vi "DisplayPanel.vi"() -> ()   [LabVIEW 2013]
uses:
  MvLVLib/MvCameraControl.lvlib
  MvLVLib/VIs/CreateGigEHandle.vi
  MvLVLib/VIs/CreateU3VHandle.vi
panel:
  out "GenTLDeviceArray":T1(array[cluster])
  out "Image":T2(plugin-control)
  out "U3VDeviceArray":T3(array[cluster])
  out "GigEDeviceArray":T4(array[cluster])
  in  "pConvertInfo In":T5
  out "PixelFormat":u32
  out "handle out":u64
  in  "handle":u64
  out "PayloadSize":u32
  out "pFrameInfoEx out":T6
  out "nHeight":u32
  out "nWidth":u32
  out "Acquisision Flag":bool
  in  "Trigger Mode":bool
  in  "Continuous":bool
  out "打开标志":bool
  in  "stop":bool
  in  "Trigger Once":bool
  in  "Stop":bool
  in  "Start":bool
  in  "Open Device":bool
  in  "Close Device":bool
  in  "error in (no error) 2":errorcluster caption="错误输入（无错误）"
  in  "Refresh Devices":bool
  in  "Device List":u16(ring)
  # "Initialize"
  # "Acquisition"
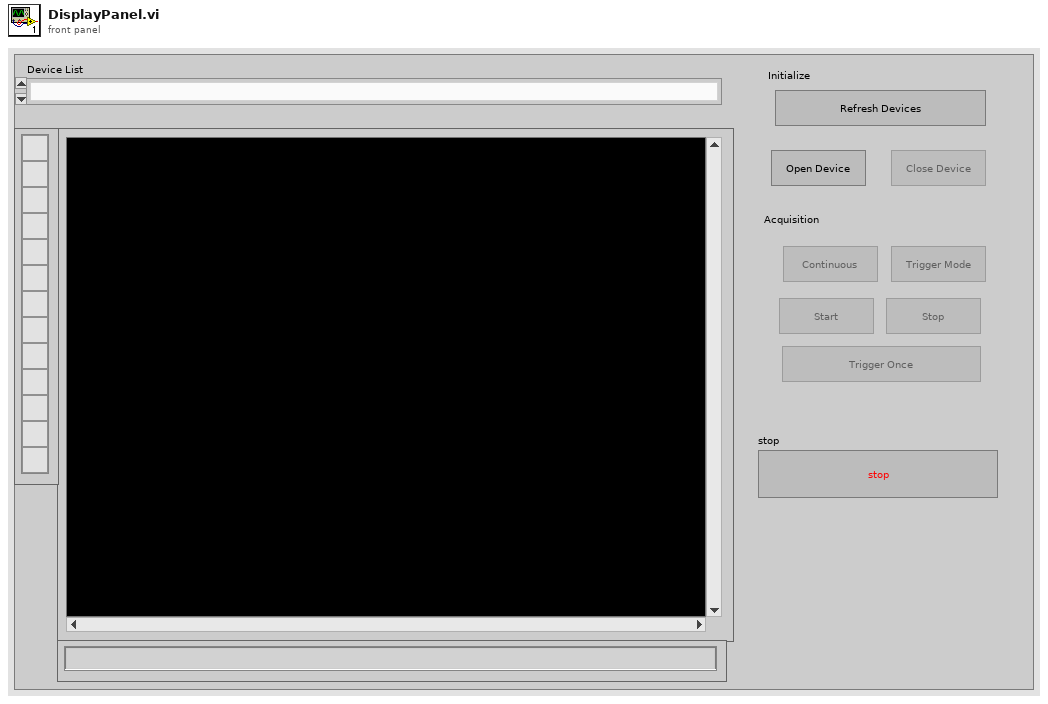
[diagram p1: front panel]
types:
  T1 = cluster{"nMajorVer":u16, "nMinorVer":u16, "nMacAddrHigh":u32, "nMacAddrLow":u32, "nTLayerType":u32, "nReserved0":u32, "nReserved1":u32, "nReserved2":u32, "nReserved3":u32, "chInterfaceID":string, "chVendorName":string, "chModelName":string, "chManufacturerInfo":string, "chDeviceVersion":string, "chSerialNumber":string, "chUserDefinedName":string, "chDeviceID":string, "nRes0":u32, "nRes1":u32, "nRes2":u32, "nRes3":u32, "nRes4":u32, "nRes5":u32, "nRes6":u32}[]
  T2 = typedef "IMAQ Image.ctl" = refnum<image>
  T3 = cluster{"nMajorVer":u16, "nMinorVer":u16, "nMacAddrHigh":u32, "nMacAddrLow":u32, "nTLayerType":u32, "nReserved0":u32, "nReserved1":u32, "nReserved2":u32, "nReserved3":u32, "CrtlInEndPoint":u8, "CrtlOutEndPoint":u8, "StreamEndPoint":u8, "EventEndPoint":u8, "idVendor":u16, "idProduct":u16, "nDeviceNumber":u32, "chDeviceGUID":string, "chVendorName":string, "chModelName":string, "chFamilyName":string, "chDeviceVersion":string, "chManufacturerName":string, "chSerialNumber":string, "chUserDefinedName":string, "nbcdUSB":u32, "nDeviceAddress":u32, "nRes0":u32, "nRes1":u32, "nResAlign":u32}[]
  T4 = cluster{"nMajorVer":u16, "nMinorVer":u16, "nMacAddrHigh":u32, "nMacAddrLow":u32, "nTLayerType":u32, "nReserved0":u32, "nReserved1":u32, "nReserved2":u32, "nReserved3":u32, "nIpCfgOption":u32, "nIpCfgCurrent":u32, "nCurrentIp":u32, "nCurrentSubNetMask":u32, "nDefaultGateWay":u32, "chManualfacturerName":string, "chModelName":string, "chDeviceVersion":string, "chManufacturerSpecificInfo":string, "chSerialNumber":string, "chUserDefinedName":string, "nNetExport":u32, "nRes0":u32, "nRes1":u32, "nRes2":u32, "nRes3":u32}[]
  T5 = cluster{"nWidth":u16, "nHeight":u16, "enSrcPixelType":u32, "nSrcDataLen":u32, "enDstPixelType":u32, "nDstLen":u32, "nDstBufferSize":u32, "nRes0":u32, "nRes1":u32, "nRes2":u32, "nRes3":u32}
  T6 = cluster{"nWidth":u16, "nHeight":u16, "enPixelType":i32, "nFrameNum":u32, "nDevTimeStampHigh":u32, "nDevTimeStampLow":u32, "nReserved0":u32, "nHostTimeStamp":i64, "nFrameLen":u32, "nSecondCount]":u32, "nCycleCount":u32, "nCycleOffset":u32, "fGain":u32, "fExposureTime":u32, "nAverageBrightness":u32, "nRed":u32, "nGreen":u32, "nBlue":u32, "nFrameCounter":u32, "nTriggerIndex":u32, "nInput":u32, "nOutput":u32, "nOffsetX":u32, "nOffsetY":u32, "nReserved[0]":u32, "nReserved[1]":u32, "nReserved[2]":u32, "nReserved[3]":u32, "nReserved[4]":u32, "nReserved[5]":u32, "nReserved[6]":u32, "nReserved[7]":u32, "nReserved[8]":u32, "nReserved[9]":u32, "nReserved[10]":u32, "nReserved[11]":u32, "nReserved[12]":u32, "nReserved[13]":u32, "nReserved[14] 10":u32, "nReserved[15] 11":u32, "nReserved[16] 12":u32, "nReserved[17] 13":u32, "nReserved[18] 14":u32, "nReserved[19] 15":u32, "nReserved[20] 16":u32, "nReserved[21] 17":u32, "nReserved[22] 18":u32, "nReserved[23] 19":u32, "nReserved[24] 20":u32, "nReserved[25] 21":u32, "nReserved[26] 22":u32, "nReserved[27] 23":u32, "nReserved[28] 24":u32, "nReserved[29] 25":u32, "nReserved[30] 26":u32, "nReserved[31] 27":u32, "nReserved[32] 28":u32, "nReserved[33] 29":u32, "nReserved[34] 30":u32, "nReserved[35] 31":u32, "nReserved[36] 32":u32, "nReserved[37] 33":u32, "nReserved[38] 34":u32, "nReserved[39] 35":u32, "nReserved[40] 36":u32}
  T7 = enum8{"Enabled", "Disabled", "Disabled and Grayed Out"}
  T8 = cluster{"nCurValue":u32, "nMax":u32, "nMin":u32, "nInc":u32, "nReserved[0]":u32, "nReserved[1]":u32, "nReserved[2]":u32, "nReserved[3]":u32}
  T9 = cluster{"nCurValue":u32, "nSupportedNum":u32, "nSupportValue":u32[], "nReserved[0]":u32, "nReserved[1]":u32, "nReserved[2]":u32, "nReserved[3]":u32}
  T10 = cluster{"nWidth":u32, "nHeight":u32, "enSrcPixelType":u32, "nSrcDataLen":u32, "enDstPixelType":u32, "nDstLen":u32, "nDstBufferSize":u32, "nRes0":u32, "nRes1":u32, "nRes2":u32, "nRes3":u32}
  T11 = typedef "Image Type" = u32
  T12 = cluster{"nMajorVer":u16, "nMinorVer":u16, "nMacAddrHigh":u32, "nMacAddrLow":u32, "nTLayerType":u32, "nReserved0":u32, "nReserved1":u32, "nReserved2":u32, "nReserved3":u32, "nIpCfgOption":u32, "nIpCfgCurrent":u32, "nCurrentIp":u32, "nCurrentSubNetMask":u32, "nDefaultGateWay":u32, "chManualfacturerName":string, "chModelName":string, "chDeviceVersion":string, "chManufacturerSpecificInfo":string, "chSerialNumber":string, "chUserDefinedName":string, "nNetExport":u32, "nRes0":u32, "nRes1":u32, "nRes2":u32, "nRes3":u32}
  T13 = cluster{"nMajorVer":u16, "nMinorVer":u16, "nMacAddrHigh":u32, "nMacAddrLow":u32, "nTLayerType":u32, "nReserved0":u32, "nReserved1":u32, "nReserved2":u32, "nReserved3":u32, "CrtlInEndPoint":u8, "CrtlOutEndPoint":u8, "StreamEndPoint":u8, "EventEndPoint":u8, "idVendor":u16, "idProduct":u16, "nDeviceNumber":u32, "chDeviceGUID":string, "chVendorName":string, "chModelName":string, "chFamilyName":string, "chDeviceVersion":string, "chManufacturerName":string, "chSerialNumber":string, "chUserDefinedName":string, "nbcdUSB":u32, "nDeviceAddress":u32, "nRes0":u32, "nRes1":u32, "nResAlign":u32}
  T14 = cluster{"nMajorVer":u16, "nMinorVer":u16, "nMacAddrHigh":u32, "nMacAddrLow":u32, "nTLayerType":u32, "nReserved0":u32, "nReserved1":u32, "nReserved2":u32, "nReserved3":u32, "chInterfaceID":string, "chVendorName":string, "chModelName":string, "chManufacturerInfo":string, "chDeviceVersion":string, "chSerialNumber":string, "chUserDefinedName":string, "chDeviceID":string, "nRes0":u32, "nRes1":u32, "nRes2":u32, "nRes3":u32, "nRes4":u32, "nRes5":u32, "nRes6":u32}
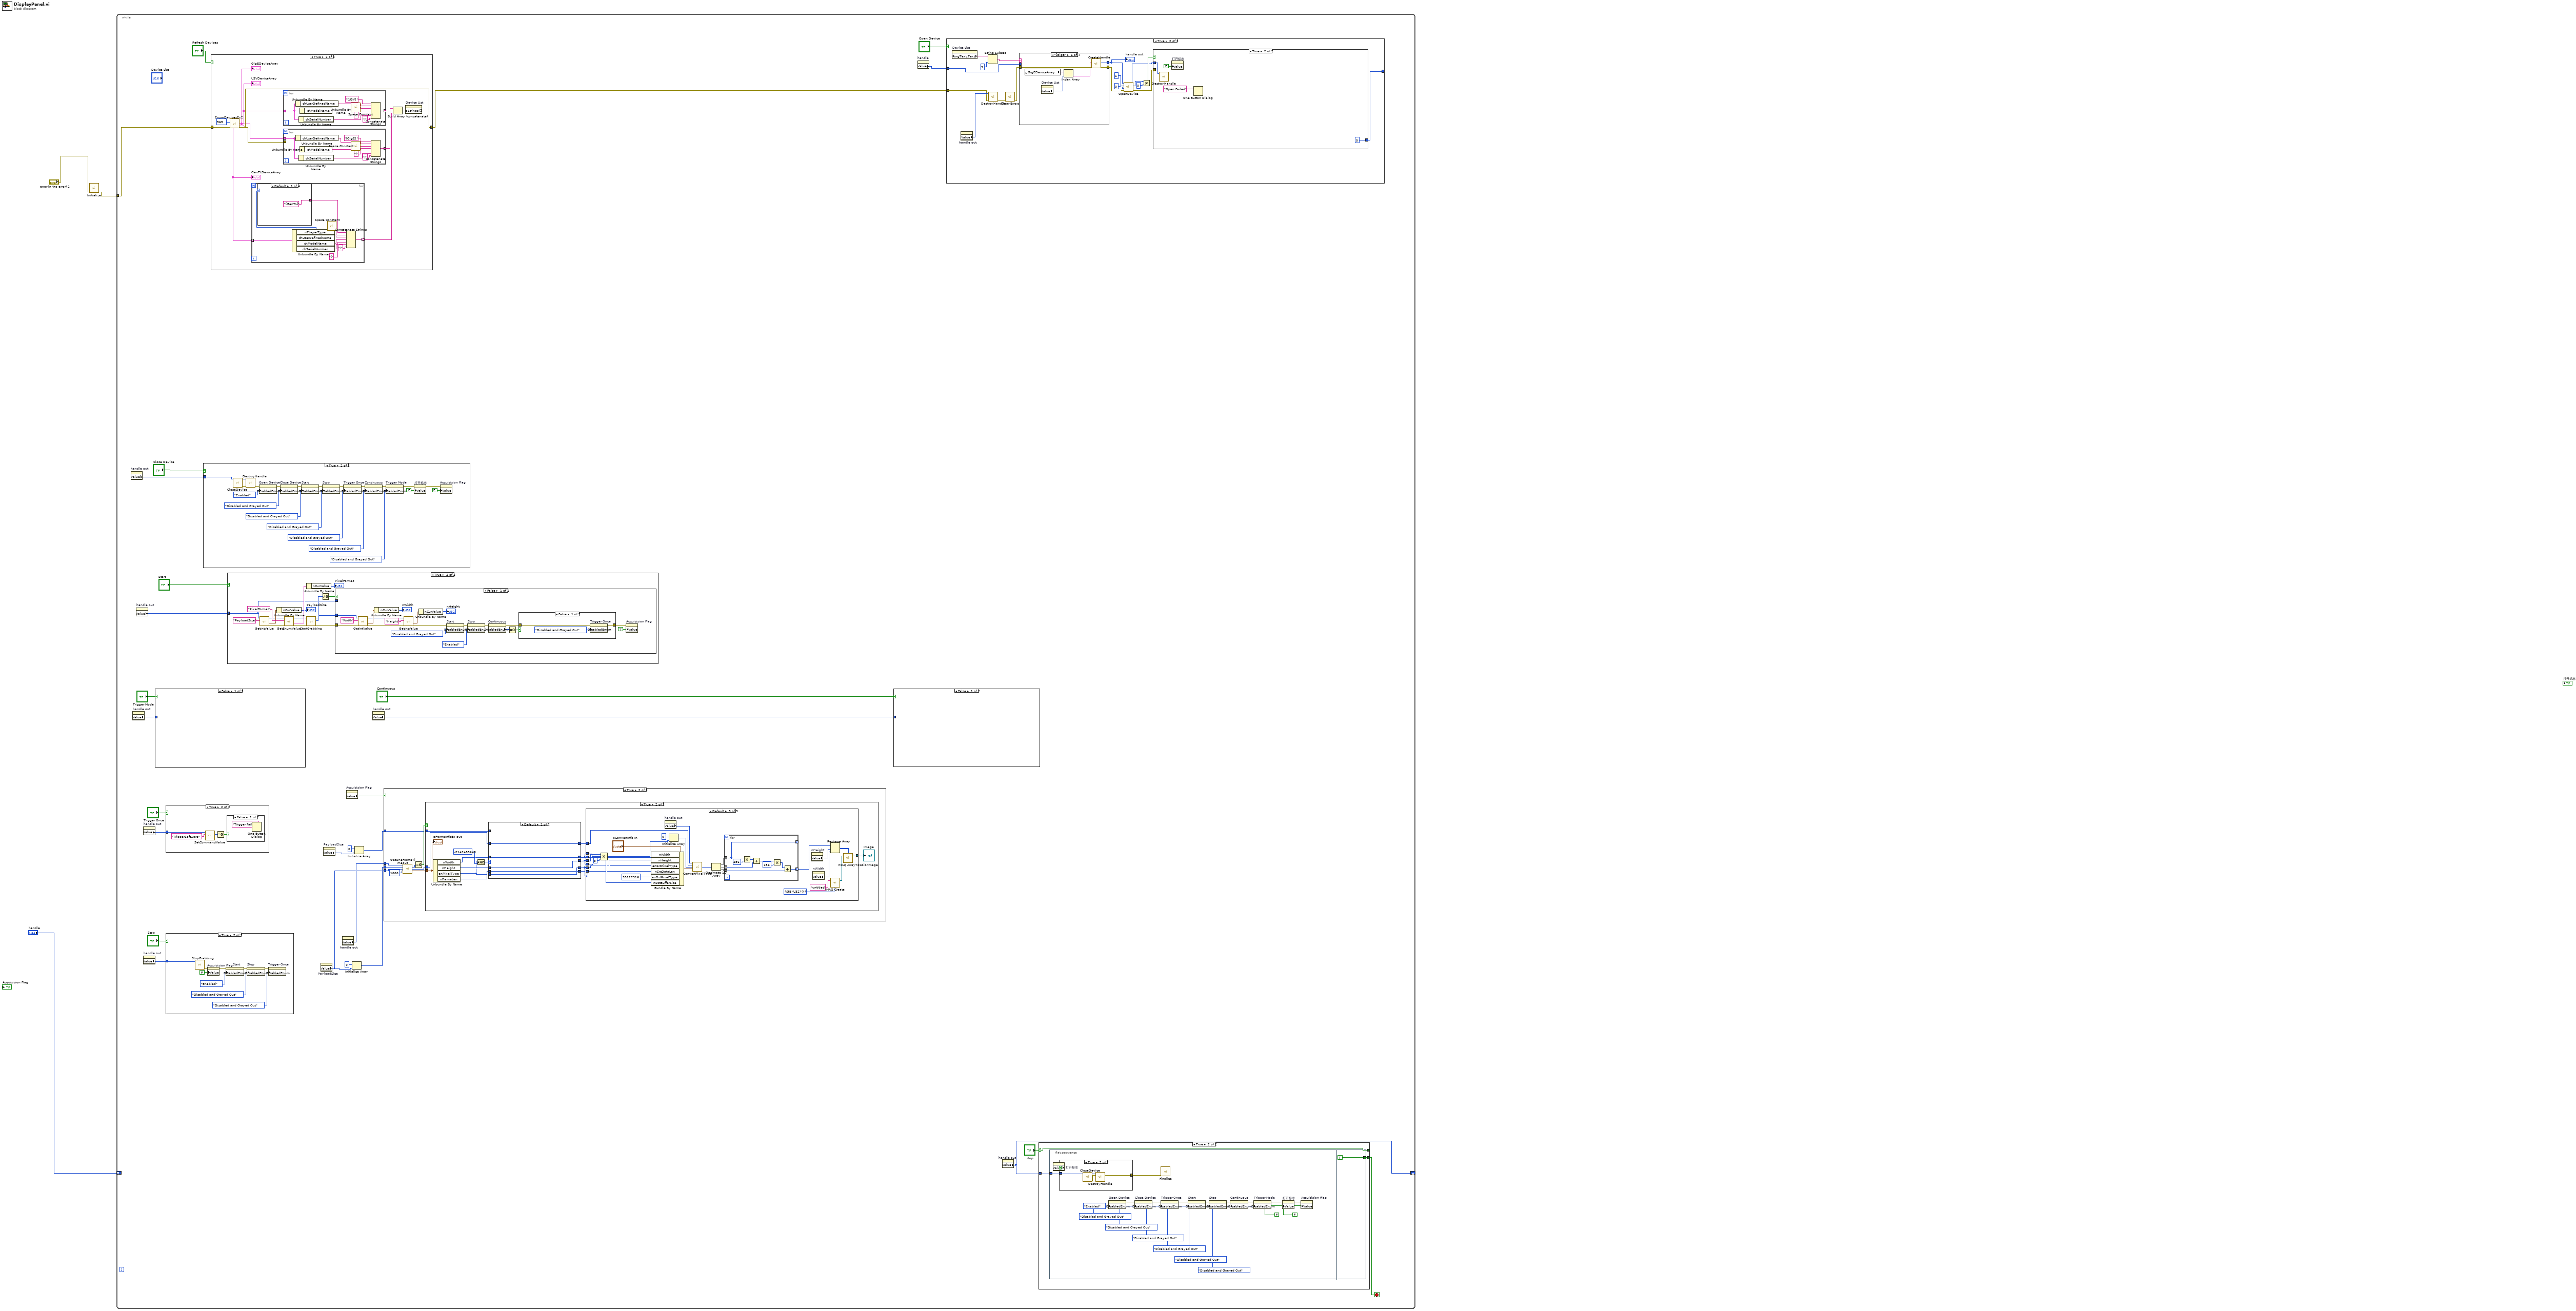
[diagram p0: block diagram]
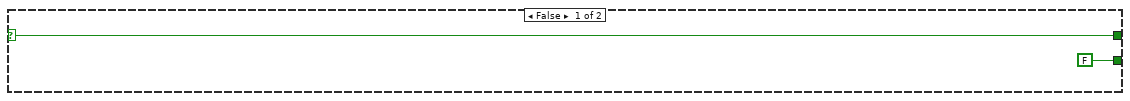
[diagram p2: hidden frame]
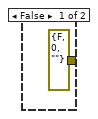
[diagram p3: hidden frame]
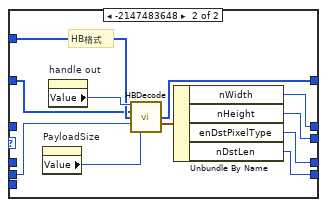
[diagram p6: hidden frame]
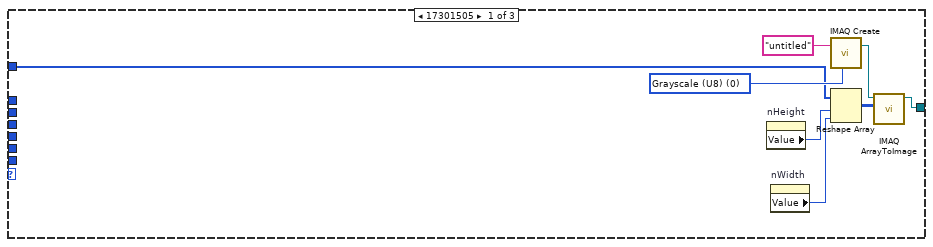
[diagram p7: hidden frame]
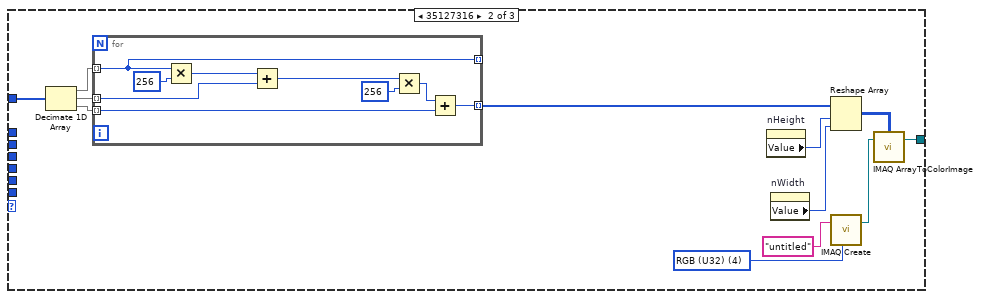
[diagram p8: hidden frame]
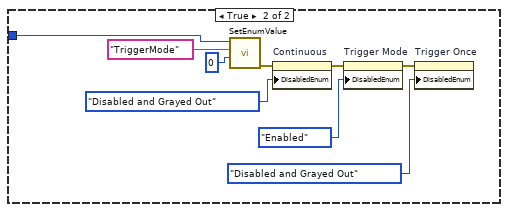
[diagram p10: hidden frame]
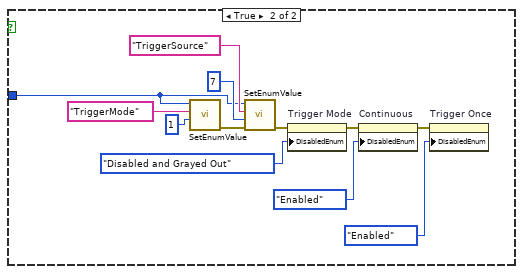
[diagram p11: hidden frame]
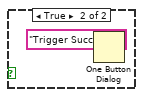
[diagram p13: hidden frame]
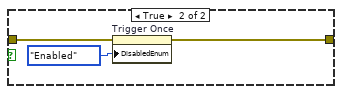
[diagram p15: hidden frame]
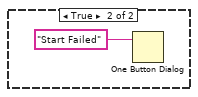
[diagram p16: hidden frame]
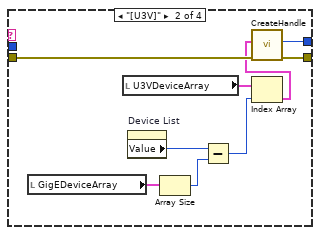
[diagram p19: hidden frame]
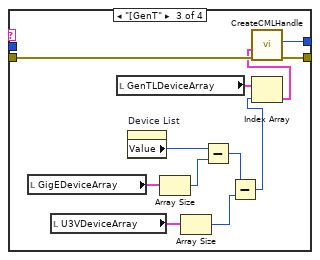
[diagram p20: hidden frame]
diagram:
  n1 = call "Initialize.vi"("error in (no error)"="error in (no error) 2") -> ("error out"=w2:errorcluster)  [unwired: 9 in, 1 out]
  n2 = while {
    shift-right: [w10] -> _
    shift-left: "handle" -> [_]
    tunnel: w2 -> [w11]
    stop <- w8 stop-if-true
    n3 = property on="handle out" class="DigNum (strict)"() -> ("Value"=w20:u64)  [unwired: 2 in, 2 out]
    n4 = property on="handle out" class="DigNum (strict)"() -> ("Value"=w15:u64)  [unwired: 2 in, 2 out]
    n5 = property on="handle out" class="DigNum (strict)"() -> ("Value"=w16:u64)  [unwired: 2 in, 2 out]
    n6 = property on="handle out" class="DigNum (strict)"() -> ("Value"=w19:u64)  [unwired: 2 in, 2 out]
    n7 = property on="handle out" class="DigNum (strict)"() -> ("Value"=w18:u64)  [unwired: 2 in, 2 out]
    n8 = case shown="False" "Trigger Mode" {
      tunnel: w15 -> [_ w186]
      frame False {
      }
      frame True {
        n9 = call "SetEnumValue.vi"("nValue"=u32 1, "strKey"="TriggerMode", "handle"=w186) -> ("error out"=w192:errorcluster)  [unwired: 6 in, 2 out]
        n10 = call "SetEnumValue.vi"("error in (no error)"=w192, "nValue"=u32 7, "strKey"="TriggerSource", "handle"=w186) -> ("error out"=w191:errorcluster)  [unwired: 5 in, 2 out]
        n11 = property on="Trigger Mode" class="Bool"(error in=w191, "DisabledEnum"=T7."Disabled and Grayed Out" ("禁用")) -> (error out=w190:errorcluster)  [unwired: 1 in, 1 out]
        n12 = property on="Continuous" class="Bool"(error in=w190, "DisabledEnum"=T7."Enabled" ("禁用")) -> (error out=w188:errorcluster)  [unwired: 1 in, 1 out]
        n13 = property on="Trigger Once" class="Bool"(error in=w188, "DisabledEnum"=T7."Enabled" ("禁用")) -> ()  [unwired: 1 in, 2 out]
      }
    }
    n14 = case shown="True" "Trigger Once" {
      tunnel: w19 -> [_ w201]
      frame False {
      }
      frame True {
        n15 = call "SetCommandValue.vi"("strValue"="TriggerSoftware", "handle"=w201) -> ("function return"=w199:i32)  [unwired: 7 in, 2 out]
        n16 = Equal To 0?(x=w199) -> (x = 0?=w198:bool)
        n17 = case shown="False" w198 {
          frame False {
            n18 = One Button Dialog(message="Trigger Failed") -> ()  [unwired: 1 in, 1 out]
          }
          frame True {
            n19 = One Button Dialog(message="Trigger Success") -> ()  [unwired: 1 in, 1 out]
          }
        }
      }
    }
    n20 = case shown="True" "Stop" {
      tunnel: w18 -> [_ w176]
      frame False {
      }
      frame True {
        n21 = call "StopGrabbing.vi"("handle"=w176) -> ("error out"=w175:errorcluster)  [unwired: 8 in, 2 out]
        n22 = property on="Acquisision Flag" class="Bool (strict)"(error in=w175, "Value"=FALSE ("采集标志")) -> (error out=w170:errorcluster)  [unwired: 1 in, 1 out]
        n23 = property on="Start" class="Bool"(error in=w170, "DisabledEnum"=T7."Enabled" ("禁用")) -> (error out=w169:errorcluster)  [unwired: 1 in, 1 out]
        n24 = property on="Stop" class="Bool"(error in=w169, "DisabledEnum"=T7."Disabled and Grayed Out" ("禁用")) -> (error out=w168:errorcluster)  [unwired: 1 in, 1 out]
        n25 = property on="Trigger Once" class="Bool"(error in=w168, "DisabledEnum"=T7."Disabled and Grayed Out" ("禁用")) -> ()  [unwired: 1 in, 2 out]
      }
    }
    n26 = case shown="True" "Close Device" {
      tunnel: w20 -> [_ w247]
      frame False {
      }
      frame True {
        n27 = call "CloseDevice.vi"("handle"=w247) -> ("error out"=w249:errorcluster, "handle out"=w246:u64)  [unwired: 8 in, 1 out]
        n28 = call "DestroyHandle.vi"("error in (no error)"=w249, "handle"=w246) -> ("error out"=w248:errorcluster)  [unwired: 8 in, 1 out]
        n29 = property on="Open Device" class="Bool"(error in=w248, "DisabledEnum"=T7."Enabled" ("禁用")) -> (error out=w262:errorcluster)  [unwired: 1 in, 1 out]
        n30 = property on="Close Device" class="Bool"(error in=w262, "DisabledEnum"=T7."Disabled and Grayed Out" ("禁用")) -> (error out=w261:errorcluster)  [unwired: 1 in, 1 out]
        n31 = property on="Start" class="Bool"(error in=w261, "DisabledEnum"=T7."Disabled and Grayed Out" ("禁用")) -> (error out=w260:errorcluster)  [unwired: 1 in, 1 out]
        n32 = property on="Stop" class="Bool"(error in=w260, "DisabledEnum"=T7."Disabled and Grayed Out" ("禁用")) -> (error out=w259:errorcluster)  [unwired: 1 in, 1 out]
        n33 = property on="Trigger Once" class="Bool"(error in=w259, "DisabledEnum"=T7."Disabled and Grayed Out" ("禁用")) -> (error out=w256:errorcluster)  [unwired: 1 in, 1 out]
        n34 = property on="Continuous" class="Bool"(error in=w256, "DisabledEnum"=T7."Disabled and Grayed Out" ("禁用")) -> (error out=w254:errorcluster)  [unwired: 1 in, 1 out]
        n35 = property on="Trigger Mode" class="Bool"(error in=w254, "DisabledEnum"=T7."Disabled and Grayed Out" ("禁用")) -> (error out=w253:errorcluster)  [unwired: 1 in, 1 out]
        n36 = property on="打开标志" class="Bool (strict)"(error in=w253, "Value"=FALSE ("打开标志")) -> (error out=w251:errorcluster)  [unwired: 1 in, 1 out]
        n37 = property on="Acquisision Flag" class="Bool (strict)"(error in=w251, "Value"=FALSE ("采集标志")) -> ()  [unwired: 1 in, 2 out]
      }
    }
    n38 = case shown="True" "Refresh Devices" {
      tunnel: [w335 w345] -> w22
      tunnel: w11 -> [w335 w344]
      frame False {
        n39 = property on="GigEDeviceArray" class="Arr (strict)" props=["Value"]() -> ()  [unwired: 2 in, 3 out]
        n40 = property on="U3VDeviceArray" class="Arr (strict)" props=["Value"]() -> ()  [unwired: 2 in, 3 out]
      }
      frame True {
        n41 = call "EnumDevicesEx2.vi"("nLayerType"=965, "error in (no error)"=w344) -> ("GigEDeviceArray"=w340:T4, "U3VDeviceArray"=w339:T3, "GenTLDevice"=w337:T1, "error out"=w345:errorcluster)  [unwired: 8 in, 2 out]
        "GigEDeviceArray" <- w340
        "U3VDeviceArray" <- w339
        "GenTLDeviceArray" <- w337
        n42 = for {
          tunnel: w337 -> [w352] mode=indexing
          tunnel: [w350] -> w336 mode=indexing
          n43 = Unbundle By Name(w352) -> ("nTLayerType"=w347:u32, "chUserDefinedName"=w355:string, "chModelName"=w349:string, "chSerialNumber"=w348:string)
          n44 = case shown="Default" w347 {
            tunnel: ["[GenTL]" ("字符串") "[GenTL CML]" ("字符串") "[GenTL CXP]" ("字符串") "[GenTL XOF]" ("字符串")] -> w346
            frame Default {
            }
            frame 128 {
            }
            frame 256 {
            }
            frame 512 {
            }
          }
          n45 = call <vilib>:"Space Constant.vi"() -> ("String"=w354:string)
          n46 = Concatenate Strings(w346, w355, w354, w349, "(" ("字符串"), w348, ")" ("字符串")) -> (w350:string)
        }
        n47 = for {
          tunnel: w339 -> [w364] mode=indexing
          tunnel: [w361] -> w342 mode=indexing
          n48 = Unbundle By Name(w364) -> ("chUserDefinedName"=w368:string)
          n49 = Unbundle By Name(w364) -> ("chSerialNumber"=w363:string)
          n50 = Unbundle By Name(w364) -> ("chModelName"=w366:string)
          n51 = call <vilib>:"Space Constant.vi"() -> ("String"=w367:string)
          n52 = Concatenate Strings("[U3V] " ("字符串"), w368, w367, w366, "(" ("字符串"), w363, ")" ("字符串")) -> (w361:string)
        }
        n53 = for {
          tunnel: w345 -> [_]
          tunnel: w340 -> [w371] mode=indexing
          tunnel: [w370] -> w343 mode=indexing
          n54 = Unbundle By Name(w371) -> ("chUserDefinedName"=w374:string)
          n55 = Unbundle By Name(w371) -> ("chSerialNumber"=w372:string)
          n56 = Unbundle By Name(w371) -> ("chModelName"=w373:string)
          n57 = call <vilib>:"Space Constant.vi"() -> ("String"=w377:string)
          n58 = Concatenate Strings("[GigE] " ("字符串"), w374, w377, w373, "(" ("字符串"), w372, ")" ("字符串")) -> (w370:string)
        }
        n59 = Build Array (concatenate)(w343, w342, w336) -> (w341:string[])
        n60 = property on="Device List" class="Ring (strict)"("Strings []"=w341) -> ()  [unwired: 2 in, 2 out]
      }
    }
    n61 = case shown="True" "Start" {
      tunnel: w16 -> [_ w208]
      frame False {
      }
      frame True {
        n62 = call "GetIntValue.vi"("strKey"="PayloadSize", "handle"=w208) -> ("error out"=w214:errorcluster, "pIntValue out"=w210:T8, "handle out"=w206:u64)  [unwired: 6 in, 1 out]
        n63 = Unbundle By Name(w210) -> ("nCurValue"=→"PayloadSize":u32)
        n64 = call "GetEnumValue.vi"("error in (no error)"=w214, "strKey"="PixelFormat", "handle"=w206) -> ("error out"=w213:errorcluster, "pEnumValue out"=w215:T9, "handle out"=w205:u64)  [unwired: 5 in, 1 out]
        n65 = Unbundle By Name(w215) -> ("nCurValue"=→"PixelFormat":u32)
        n66 = call "StartGrabbing.vi"("error in (no error)"=w213, "handle"=w205) -> ("error out"=w212:errorcluster, "function return"=w218:i32, "handle out"=w204:u64)  [unwired: 7 in]
        n67 = Not Equal To 0?(x=w218) -> (x != 0?=w217:bool)
        n68 = case shown="False" w217 {
          tunnel: w208 -> [_ _]
          tunnel: w212 -> [w221 _]
          tunnel: w204 -> [w220 _]
          frame False {
            n69 = call "GetIntValue.vi"("error in (no error)"=w221, "strKey"="Width", "handle"=w220) -> ("error out"=w228:errorcluster, "pIntValue out"=w222:T8, "handle out"=w219:u64)  [unwired: 5 in, 1 out]
            n70 = Unbundle By Name(w222) -> ("nCurValue"=→"nWidth":u32)
            n71 = call "GetIntValue.vi"("error in (no error)"=w228, "strKey"="Height", "handle"=w219) -> ("error out"=w227:errorcluster, "pIntValue out"=w225:T8)  [unwired: 5 in, 2 out]
            n72 = Unbundle By Name(w225) -> ("nCurValue"=→"nHeight":u32)
            n73 = property on="Start" class="Bool"(error in=w227, "DisabledEnum"=T7."Disabled and Grayed Out" ("禁用")) -> (error out=w237:errorcluster)  [unwired: 1 in, 1 out]
            n74 = property on="Stop" class="Bool"(error in=w237, "DisabledEnum"=T7."Enabled" ("禁用")) -> (error out=w223:errorcluster)  [unwired: 1 in, 1 out]
            n75 = property on="Continuous" class="Bool"(error in=w223) -> (error out=w233:errorcluster, "DisabledEnum"=w234:T7)  [unwired: 1 in, 1 out]
            n76 = Equal To 0?(x=w234) -> (x = 0?=w235:bool)
            n77 = case shown="False" w235 {
              tunnel: w233 -> [w240 w243]
              tunnel: [w239 w242] -> w232
              frame False {
                n78 = property on="Trigger Once" class="Bool"(error in=w240, "DisabledEnum"=T7."Disabled and Grayed Out" ("禁用")) -> (error out=w239:errorcluster)  [unwired: 1 in, 1 out]
              }
              frame True {
                n79 = property on="Trigger Once" class="Bool"(error in=w243, "DisabledEnum"=T7."Enabled" ("禁用")) -> (error out=w242:errorcluster)  [unwired: 1 in, 1 out]
              }
            }
            n80 = property on="Acquisision Flag" class="Bool (strict)"(error in=w232, "Value"=TRUE ("采集标志")) -> ()  [unwired: 1 in, 2 out]
          }
          frame True {
            n81 = One Button Dialog(message="Start Failed") -> ()  [unwired: 1 in, 1 out]
          }
        }
      }
    }
    n82 = property on="PayloadSize" class="DigNum (strict)"() -> ("Value"=w7:u32)  [unwired: 2 in, 2 out]
    n83 = property on="PayloadSize" class="DigNum (strict)"() -> ("Value"=w6:u32)  [unwired: 2 in, 2 out]
    n84 = property on="handle out" class="DigNum (strict)"() -> ("Value"=w17:u64)  [unwired: 2 in, 2 out]
    n85 = property on="Acquisision Flag" class="Bool (strict)"() -> ("Value"=w23:bool)  [unwired: 2 in, 2 out]
    n86 = Initialize Array(u8 0 ("元素"), w7) -> (w12:u8[])
    n87 = Initialize Array(u8 0 ("元素"), w6) -> (w4:u8[])
    n88 = property on="handle out" class="DigNum (strict)"() -> ("Value"=w14:u64)  [unwired: 2 in, 2 out]
    n89 = case shown="True" w23 {
      tunnel: w17 -> [_ w69]
      tunnel: w12 -> [_ w68]
      tunnel: w7 -> [_ w67]
      tunnel: w4 -> [_ w63]
      frame False {
      }
      frame True {
        n90 = call "GetOneFrameTimeout.vi"("handle"=w69, "pData"=w68, "nDataSize"=w67, "nMsec"=1000) -> ("function return"=w66:i32, "pData Out"=w65:u8[], "pFrameInfoEx out"=w64:T6)  [unwired: 7 in, 2 out]
        n91 = Equal To 0?(x=w66) -> (x = 0?=w71:bool)
        n92 = case shown="True" w71 {
          tunnel: w65 -> [_ w81]
          tunnel: w64 -> [_ w85]
          tunnel: w63 -> [_ w82]
          frame False {
          }
          frame True {
            n93 = Unbundle By Name(w85) -> ("nWidth"=w74:u16, "nHeight"=w73:u16, "enPixelType"=w72:i32, "nFrameLen"=w80:u32)
            n94 = Compound Arithmetic op=AND(w72, -2147483648 ("value")) -> (w83:i32)
            n95 = case shown="Default" w83 {
              tunnel: w82 -> [_ w101]
              tunnel: w81 -> [w91 w100]
              tunnel: w80 -> [w88 w99]
              tunnel: [w91 w96] -> w79
              tunnel: [w90 w95] -> w78
              tunnel: [w89 w94] -> w77
              tunnel: [w87 w93] -> w76
              tunnel: [w88 w92] -> w75
              tunnel: w74 -> [w90 _]
              tunnel: w73 -> [w89 _]
              tunnel: w72 -> [w87 _]
              frame Default {
              }
              frame -2147483648 {
                # "HB格式"
                n96 = property on="PayloadSize" class="DigNum (strict)"() -> ("Value"=w98:u32)  [unwired: 2 in, 2 out]
                n97 = property on="handle out" class="DigNum (strict)"() -> ("Value"=w102:u64)  [unwired: 2 in, 2 out]
                n98 = call "HBDecode.vi"("handle"=w102, "pSrcData"=w100, "pDstBuf In"=w101, "SrcDataLen"=w99, "DstBufferSize"=w98) -> ("pDstBuf Out"=w96:u8[], "pHBDecode Out"=w97:T10)  [unwired: 6 in, 3 out]
                n99 = Unbundle By Name(w97) -> ("nWidth"=w95:u32, "nHeight"=w94:u32, "enDstPixelType"=w93:u32, "nDstLen"=w92:u32)
              }
            }
            n100 = case shown="Default" w76 {
              tunnel: w79 -> [w103 w114 w132]
              tunnel: w77 -> [_ _ w153]
              tunnel: w78 -> [_ _ w152]
              tunnel: [w104 w113 w137] -> w86
              tunnel: w78 -> [_ _ w136]
              tunnel: w77 -> [_ _ w135]
              tunnel: w76 -> [_ _ w134]
              tunnel: w75 -> [_ _ w133]
              frame 17301505 {
                w110 = T11 0 items=["Grayscale (U8)", "Grayscale (I16)", "Grayscale (SGL)", "Complex (CSG)", "RGB (U32)", "HSL (U32)", "RGB (U64)", "Grayscale (U16)"] ("Image Type")
                n101 = property on="nHeight" class="DigNum (strict)"() -> ("Value"=w106:u32)  [unwired: 2 in, 2 out]
                n102 = property on="nWidth" class="DigNum (strict)"() -> ("Value"=w105:u32)  [unwired: 2 in, 2 out]
                n103 = call "IMAQ Create"("Image Name"="untitled", "Image Type"=w110) -> ("New Image"=w108:T2)  [unwired: 3 in, 1 out]
                n104 = Reshape Array(w103, w106, w105) -> (w107:u8[][])
                n105 = call "IMAQ ArrayToImage"("Image Pixels (U8)"=w107, "Image"=w108) -> ("Image Out"=w104:T2)  [unwired: 8 in, 1 out]
              }
              frame 35127316 {
                w122 = T11 4 items=["Grayscale (U8)", "Grayscale (I16)", "Grayscale (SGL)", "Complex (CSG)", "RGB (U32)", "HSL (U32)", "RGB (U64)", "Grayscale (U16)"] ("Image Type")
                n106 = Decimate 1D Array(w114) -> (w115:u8[], w116:u8[], w117:u8[])
                n107 = for {
                  tunnel: w115 -> [w123] mode=indexing
                  tunnel: w116 -> [w129] mode=indexing
                  tunnel: w117 -> [w125] mode=indexing
                  tunnel: [w124] -> w118 mode=indexing
                  tunnel: [w123] -> _ mode=indexing
                  n108 = Multiply(x=w123, y=256) -> (x*y=w130:i32)
                  n109 = Add(x=w130, y=w129) -> (x+y=w128:i32)
                  n110 = Multiply(x=w128, y=256) -> (x*y=w126:i32)
                  n111 = Add(x=w126, y=w125) -> (x+y=w124:i32)
                }
                n112 = property on="nHeight" class="DigNum (strict)"() -> ("Value"=w112:u32)  [unwired: 2 in, 2 out]
                n113 = property on="nWidth" class="DigNum (strict)"() -> ("Value"=w111:u32)  [unwired: 2 in, 2 out]
                n114 = Reshape Array(w118, w112, w111) -> (w119:i32[][])
                n115 = call "IMAQ Create"("Image Name"="untitled", "Image Type"=w122) -> ("New Image"=w120:T2)  [unwired: 3 in, 1 out]
                n116 = call "IMAQ ArrayToColorImage"("Image Pixels (U32)"=w119, "Image"=w120) -> ("Image Out"=w113:T2)  [unwired: 3 in, 1 out]
              }
              frame Default {
                w148 = T11 4 items=["Grayscale (U8)", "Grayscale (I16)", "Grayscale (SGL)", "Complex (CSG)", "RGB (U32)", "HSL (U32)", "RGB (U64)", "Grayscale (U16)"] ("Image Type")
                n117 = Compound Arithmetic op=MULTIPLY(w153, w152, u32 3 ("值")) -> (w150:u32)
                n118 = Bundle By Name(cluster="pConvertInfo In", "nWidth"=w136, "nHeight"=w135, "enSrcPixelType"=w134, "nSrcDataLen"=w133, "enDstPixelType"=u32 35127316, "nDstBufferSize"=w150) -> (w149:T5)
                n119 = property on="handle out" class="DigNum (strict)"() -> ("Value"=w156:u64)  [unwired: 2 in, 2 out]
                n120 = Initialize Array(u8 0 ("元素"), w150) -> (w155:u8[])
                n121 = call "ConvertPixelType.vi"("handle"=w156, "pSrcData"=w132, "pDstBuf In"=w155, "pConvertInfo In"=w149) -> ("pDstBuf Out"=w140:u8[])  [unwired: 7 in, 4 out]
                n122 = Decimate 1D Array(w140) -> (w141:u8[], w142:u8[], w143:u8[])
                n123 = for {
                  tunnel: w141 -> [w159] mode=indexing
                  tunnel: w142 -> [w165] mode=indexing
                  tunnel: w143 -> [w161] mode=indexing
                  tunnel: [w160] -> w144 mode=indexing
                  tunnel: [w159] -> _ mode=indexing
                  n124 = Multiply(x=w159, y=256) -> (x*y=w166:i32)
                  n125 = Add(x=w166, y=w165) -> (x+y=w164:i32)
                  n126 = Multiply(x=w164, y=256) -> (x*y=w162:i32)
                  n127 = Add(x=w162, y=w161) -> (x+y=w160:i32)
                }
                n128 = property on="nHeight" class="DigNum (strict)"() -> ("Value"=w139:u32)  [unwired: 2 in, 2 out]
                n129 = property on="nWidth" class="DigNum (strict)"() -> ("Value"=w138:u32)  [unwired: 2 in, 2 out]
                n130 = Reshape Array(w144, w139, w138) -> (w145:i32[][])
                n131 = call "IMAQ Create"("Image Name"="untitled", "Image Type"=w148) -> ("New Image"=w146:T2)  [unwired: 3 in, 1 out]
                n132 = call "IMAQ ArrayToColorImage"("Image Pixels (U32)"=w145, "Image"=w146) -> ("Image Out"=w137:T2)  [unwired: 3 in, 1 out]
              }
            }
            "Image" <- w86
            "pFrameInfoEx out" <- w85
          }
        }
      }
    }
    n133 = case shown="False" "Continuous" {
      tunnel: w14 -> [_ w177]
      frame False {
      }
      frame True {
        n134 = call "SetEnumValue.vi"("nValue"=u32 0, "strKey"="TriggerMode", "handle"=w177) -> ("error out"=w178:errorcluster)  [unwired: 6 in, 2 out]
        n135 = property on="Continuous" class="Bool"(error in=w178, "DisabledEnum"=T7."Disabled and Grayed Out" ("禁用")) -> (error out=w182:errorcluster)  [unwired: 1 in, 1 out]
        n136 = property on="Trigger Mode" class="Bool"(error in=w182, "DisabledEnum"=T7."Enabled" ("禁用")) -> (error out=w180:errorcluster)  [unwired: 1 in, 1 out]
        n137 = property on="Trigger Once" class="Bool"(error in=w180, "DisabledEnum"=T7."Disabled and Grayed Out" ("禁用")) -> ()  [unwired: 1 in, 2 out]
      }
    }
    n138 = property on="handle" class="DigNum (strict)"() -> ("Value"=w21:u64)  [unwired: 2 in, 2 out]
    n139 = case shown="True" "Open Device" {
      tunnel: [w267 w278] -> _
      tunnel: w21 -> [w267 w268]
      tunnel: w22 -> [_ w272]
      frame False {
      }
      frame True {
        n140 = property on="Device List" class="Ring (strict)"() -> ("RingText.Text"=w277:string)  [unwired: 2 in, 2 out]
        n141 = property on="handle out" class="DigNum (strict)"() -> ("Value"=w273:u64)  [unwired: 2 in, 2 out]
        n142 = String Subset(string=w277, length (rest)=5 ("长度（剩余）")) -> (substring=w269:string)  [unwired: 1 in]
        n143 = call "DestroyHandle.vi"("error in (no error)"=w272, "handle"=w273) -> ("error out"=w271:errorcluster)  [unwired: 8 in, 1 out]
        n144 = call <vilib>:"Clear Errors.vi"("error in (no error)"=w271) -> ("error out"=w270:errorcluster)  [unwired: 5 in, 1 out]
        n145 = case shown="\"[GigE\"" w269 {
          tunnel: [w289 w296 w309 w314] -> w283
          tunnel: [w288 w295 w308 w313] -> w279
          tunnel: w270 -> [w290 w297 w310 w314]
          tunnel: w268 -> [_ _ _ w313]
          frame "[GigE" {
            n146 = local read "GigEDeviceArray"() -> (w287:T4)
            n147 = property on="Device List" class="Ring (strict)"() -> ("Value"=w291:u16)  [unwired: 2 in, 2 out]
            n148 = Index Array(array=w287, index=w291) -> (element=w286:T12)
            n149 = call-poly "CreateHandle.vi"("error in (no error)"=w290, "GigEDevice"=w286) -> ("error out"=w289:errorcluster, "handle"=w288:u64)  [unwired: 6 in, 1 out]
          }
          frame "[U3V]" {
            n150 = local read "GigEDeviceArray"() -> (w293:T4)
            n151 = local read "U3VDeviceArray"() -> (w294:T3)
            n152 = property on="Device List" class="Ring (strict)"() -> ("Value"=w300:u16)  [unwired: 2 in, 2 out]
            n153 = Array Size(array=w293) -> (size(s)=w299:i32)
            n154 = Subtract(x=w300, y=w299) -> (x-y=w298:i32)
            n155 = Index Array(array=w294, index=w298) -> (element=w292:T13)
            n156 = call-poly "CreateHandle.vi"("error in (no error)"=w297, "U3VDevice"=w292) -> ("error out"=w296:errorcluster, "handle"=w295:u64)  [unwired: 6 in, 1 out]
          }
          frame "[GenT" {
            n157 = local read "GigEDeviceArray"() -> (w306:T4)
            n158 = local read "U3VDeviceArray"() -> (w305:T3)
            n159 = local read "GenTLDeviceArray"() -> (w307:T1)
            n160 = property on="Device List" class="Ring (strict)"() -> ("Value"=w312:u16)  [unwired: 2 in, 2 out]
            n161 = Array Size(array=w306) -> (size(s)=w311:i32)
            n162 = Array Size(array=w305) -> (size(s)=w303:i32)
            n163 = Subtract(x=w312, y=w311) -> (x-y=w304:i32)
            n164 = Subtract(x=w304, y=w303) -> (x-y=w302:i32)
            n165 = Index Array(array=w307, index=w302) -> (element=w301:T14)
            n166 = call "CreateCMLHandle.vi"("error in (no error)"=w310, "GenTLCMLDevice"=w301) -> ("error out"=w309:errorcluster, "handle"=w308:u64)  [unwired: 6 in, 1 out]
          }
          frame Default {
          }
        }
        "handle out" <- w279
        n167 = call "OpenDevice.vi"("error in (no error)"=w283, "nSwitchoverKey"=u16 0, "nAccessMode"=u32 1, "handle"=w279) -> ("error out"=w280:errorcluster, "return"=w275:i32, "handle out"=w274:u64)  [unwired: 5 in]
        n168 = Not Equal?(x=w275, y=0) -> (x != y?=w284:bool)
        n169 = case shown="True" w284 {
          tunnel: w274 -> [w315 w332]
          tunnel: w280 -> [w316 _]
          tunnel: [w315 u64 0 ("handle")] -> w278
          frame False {
            n170 = call "SetEnumValue.vi"("error in (no error)"=w316, "nValue"=u32 0, "strKey"="TriggerMode", "handle"=w315) -> ("error out"=w327:errorcluster)  [unwired: 5 in, 2 out]
            n171 = property on="Start" class="Bool"(error in=w327, "DisabledEnum"=T7."Enabled" ("禁用")) -> (error out=w325:errorcluster)  [unwired: 1 in, 1 out]
            n172 = property on="Open Device" class="Bool"(error in=w325, "DisabledEnum"=T7."Disabled and Grayed Out" ("禁用")) -> (error out=w324:errorcluster)  [unwired: 1 in, 1 out]
            n173 = property on="Close Device" class="Bool"(error in=w324, "DisabledEnum"=T7."Enabled" ("禁用")) -> (error out=w321:errorcluster)  [unwired: 1 in, 1 out]
            n174 = property on="Trigger Mode" class="Bool"(error in=w321, "DisabledEnum"=T7."Enabled" ("禁用")) -> (error out=w319:errorcluster)  [unwired: 1 in, 1 out]
            n175 = property on="Continuous" class="Bool"(error in=w319, "DisabledEnum"=T7."Disabled and Grayed Out" ("禁用")) -> (error out=w317:errorcluster)  [unwired: 1 in, 1 out]
            n176 = property on="打开标志" class="Bool (strict)"(error in=w317, "Value"=TRUE ("布尔")) -> ()  [unwired: 1 in, 2 out]
          }
          frame True {
            n177 = call "DestroyHandle.vi"("handle"=w332) -> ()  [unwired: 9 in, 2 out]
            n178 = property on="打开标志" class="Bool (strict)"("Value"=FALSE) -> ()  [unwired: 2 in, 2 out]
            n179 = One Button Dialog(message="Open Failed") -> ()  [unwired: 1 in, 1 out]
          }
        }
      }
    }
    n180 = property on="handle out" class="DigNum (strict)"() -> ("Value"=w10:u64)  [unwired: 2 in, 2 out]
    n181 = case shown="True" "stop" {
      selector: "stop" -> [w33 w36]
      tunnel: [w33 w36] -> _
      tunnel: w10 -> [_ w35]
      tunnel: [FALSE w34] -> w8
      frame False {
      }
      frame True {
        n182 = flat-sequence {
          tunnel: w35 -> [w38]
          tunnel: [TRUE] -> w34
          frame #0 {
            n183 = property on="打开标志" class="Bool (strict)"() -> ("Value"=w43:bool)  [unwired: 2 in, 2 out]
            n184 = case shown="True" w43 {
              tunnel: w38 -> [_ w59]
              tunnel: [errorcluster {"status"=FALSE, "code"=0, "source"=""} ("error out") w58] -> w37
              frame False {
              }
              frame True {
                n185 = call "CloseDevice.vi"("handle"=w59) -> ("error out"=w61:errorcluster, "handle out"=w60:u64)  [unwired: 8 in, 1 out]
                n186 = call "DestroyHandle.vi"("error in (no error)"=w61, "handle"=w60) -> ("error out"=w58:errorcluster)  [unwired: 8 in, 1 out]
              }
            }
            n187 = property on="Open Device" class="Bool"("DisabledEnum"=T7."Enabled" ("禁用")) -> (error out=w51:errorcluster)  [unwired: 2 in, 1 out]
            n188 = property on="Close Device" class="Bool"(error in=w51, "DisabledEnum"=T7."Disabled and Grayed Out" ("禁用")) -> (error out=w50:errorcluster)  [unwired: 1 in, 1 out]
            n189 = call "Finalize.vi"("error in (no error)"=w37) -> ()  [unwired: 9 in, 2 out]
            n190 = property on="Trigger Once" class="Bool"(error in=w50, "DisabledEnum"=T7."Disabled and Grayed Out" ("禁用")) -> (error out=w49:errorcluster)  [unwired: 1 in, 1 out]
            n191 = property on="Start" class="Bool"(error in=w49, "DisabledEnum"=T7."Disabled and Grayed Out" ("禁用")) -> (error out=w48:errorcluster)  [unwired: 1 in, 1 out]
            n192 = property on="Stop" class="Bool"(error in=w48, "DisabledEnum"=T7."Disabled and Grayed Out" ("禁用")) -> (error out=w47:errorcluster)  [unwired: 1 in, 1 out]
            n193 = property on="Continuous" class="Bool"(error in=w47, "DisabledEnum"=T7."Disabled and Grayed Out" ("禁用")) -> (error out=w45:errorcluster)  [unwired: 1 in, 1 out]
            n194 = property on="Trigger Mode" class="Bool"(error in=w45, "DisabledEnum"=T7."Disabled and Grayed Out" ("禁用")) -> (error out=w40:errorcluster)  [unwired: 1 in, 1 out]
            n195 = property on="打开标志" class="Bool (strict)"(error in=w40, "Value"=FALSE ("打开标志")) -> (error out=w39:errorcluster)  [unwired: 1 in, 1 out]
            n196 = property on="Acquisision Flag" class="Bool (strict)"(error in=w39, "Value"=FALSE ("采集标志")) -> ()  [unwired: 1 in, 2 out]
          }
          frame #1 {
          }
        }
      }
    }
  }
